vi "FFT1D_CuLab.vi"(7 "Iteration":i32, 11 "samples":i32=128) -> (3 "Results(s)":dbl format="%.8f")   [LabVIEW 2020]
uses:
  <vilib>/Analysis/NI_AALBase.lvlib
  <vilib>/Ngene/CuLab - GPU Accelerated Toolkit/Toolkit/CuLab.lvlib
  <vilib>/Ngene/CuLab - GPU Accelerated Toolkit/Toolkit/Low_Level/Tensor_Classes/T_Children/T1D/T1D_Children/T1D_CSG/Create.vi
  <vilib>/Ngene/CuLab - GPU Accelerated Toolkit/Toolkit/Low_Level/Tensor_Classes/T_Children/T1D/T1D_Children/T1D_CSG/T1D_CSG.lvclass
  9db68642-0dcb-498b-b44a-62aa3c0a4411.vi
  65ef9bab-b20b-4f39-8830-9ccf3097e1d2.vi
  <vilib>/Ngene/CuLab - GPU Accelerated Toolkit/Toolkit/Low_Level/Tensor_Classes/T_Children/T1D/T1D_Children/T1D_CSG/Pull.vi
  <vilib>/Ngene/CuLab - GPU Accelerated Toolkit/Toolkit/Low_Level/Tensor_Classes/T_Children/T1D/T1D_Children/T1D_CSG/Push.vi
  <vilib>/Ngene/CuLab - GPU Accelerated Toolkit/Toolkit/API/Signal Processing/Transforms/CU_FFT/T1D/CU_FFT_T1D_C2C.vi
panel:
  out "error out":errorcluster
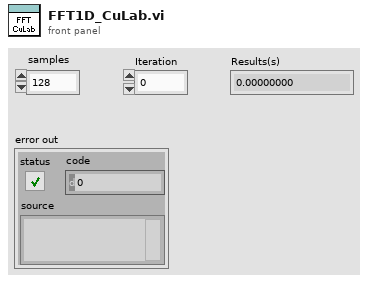
[diagram p1: front panel]
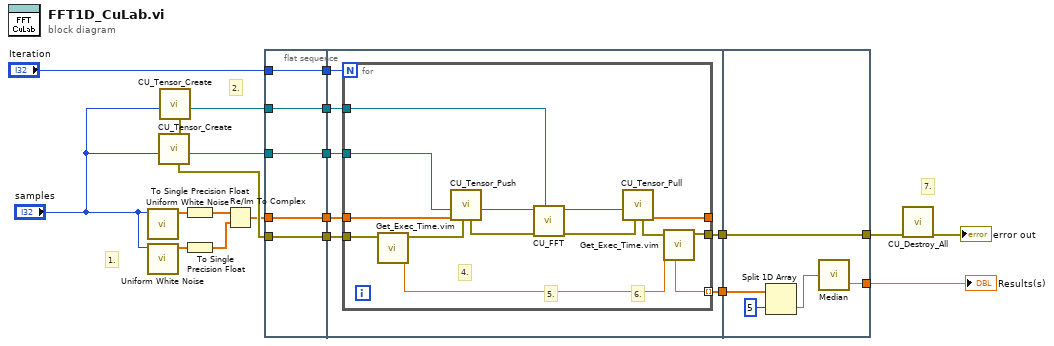
[diagram p0: block diagram]
diagram:
  # "7."
  # "2."
  # "1."
  n1 = call <vilib>:"Uniform White Noise.vi"("samples"="samples") -> ("uniform white noise"=w12:dbl[])  [unwired: 9 in, 1 out]
  n2 = call <vilib>:"Uniform White Noise.vi"("samples"="samples") -> ("uniform white noise"=w5:dbl[])  [unwired: 9 in, 1 out]
  n3 = call-poly <vilib>:"CU_Tensor_Create.vi"("Length"="samples") -> ("T1D_CSG out"=w11:refnum<class "T1D_CSG.lvclass">, "error out"=w9:errorcluster)  [unwired: 9 in]
  n4 = call-poly <vilib>:"CU_Tensor_Create.vi"("error in (no error)"=w9, "Length"="samples") -> ("T1D_CSG out"=w13:refnum<class "T1D_CSG.lvclass">, "error out"=w8:errorcluster)  [unwired: 8 in]
  n5 = To Single Precision Float(number=w12) -> (single precision float=w10:sgl[])
  n6 = To Single Precision Float(number=w5) -> (single precision float=w4:sgl[])
  n7 = Re/Im To Complex(1:w4, 2:w10) -> (0:w3:csg[])
  n8 = flat-sequence {
    tunnel: w8 -> [w22]
    tunnel: w3 -> [w23]
    tunnel: "Iteration" -> [w24]
    tunnel: w11 -> [w25]
    tunnel: w13 -> [w26]
    tunnel: [w26] -> w20
    tunnel: [w25] -> w19
    tunnel: [w24] -> w18
    tunnel: [w23] -> w17
    tunnel: [w22] -> w16
    tunnel: [w29] -> w15
    tunnel: w20 -> [w33]
    tunnel: w19 -> [w32]
    tunnel: w18 -> [w28]
    tunnel: w17 -> [w31]
    tunnel: w16 -> [w30]
    tunnel: [w27] -> w14
    tunnel: [w52] -> w7
    tunnel: w15 -> [w52]
    tunnel: [w48] -> w6
    tunnel: w14 -> [w51]
    frame #0 {
    }
    frame #1 {
      n9 = for {
        N: w28 -> [_]
        tunnel: w31 -> [w35]
        tunnel: w33 -> [w43]
        tunnel: w32 -> [w45]
        tunnel: w30 -> [w37]
        tunnel: [w38] -> w29
        tunnel: [w40] -> w27 mode=indexing
        tunnel: [w34] -> _
        # "6."
        # "5."
        # "4."
        n10 = call "Get_Exec_Time.vim"("error in (no error)"=w37) -> ("T(n)"=w41:dbl, "error out"=w36:errorcluster)  [unwired: 6 in, 1 out]
        n11 = call-poly <vilib>:"CU_Tensor_Push.vi"("error in (no error)"=w36, "CPU_Data_1D_CSG"=w35, "T1D_CSG in"=w43) -> ("T1D_CSG out"=w47:refnum<class "T1D_CSG.lvclass">, "error out"=w46:errorcluster)  [unwired: 7 in]
        n12 = call-poly <vilib>:"CU_FFT.vi"("FFT {X} dest"=w45, "error in"=w46, "X"=w47) -> ("error out"=w44:errorcluster, "FFT {X}"=w42:refnum<class "T1D_CSG.lvclass">)  [unwired: 7 in]
        n13 = call-poly <vilib>:"CU_Tensor_Pull.vi"("error in (no error)"=w44, "T1D_CSG in"=w42) -> ("Dest out"=w34:csg[], "error out"=w39:errorcluster)  [unwired: 7 in, 1 out]
        n14 = call "Get_Exec_Time.vim"("T(n-1)"=w41, "error in (no error)"=w39) -> ("error out"=w38:errorcluster, "dT"=w40:dbl)  [unwired: 5 in, 1 out]
      }
    }
    frame #2 {
      n15 = Split 1D Array(array=w51, index=5) -> (second subarray=w49:dbl[])  [unwired: 1 out]
      n16 = call <vilib>:"Median.vi"("X"=w49) -> ("median"=w48:dbl)  [unwired: 1 out]
    }
  }
  n17 = call <vilib>:"CU_Destroy_All.vi"("error in"=w7) -> ("error out"=→"error out":errorcluster)  [unwired: 10 in]
  "Results(s)" <- w6
